vi "EventstringCounter.vi"(3 "error in":errorcluster, 4 "Reset Count":bool, 5 "Increment":bool) -> (0 "error out":errorcluster, 2 "Count":u32)   [LabVIEW 2011]
doc: "Keeps count of anything you want. In this case it is meant to keep track of the number of eventstrings we've sent.\n\nSo you should call this with \"Reset Count\" = TRUE in the initialization code, and then with \"Increment\" = TRUE every time you send an eventstring. Then \"Count\" will return the total number of eventstrings sent.\n\nNo error handling happens; the error in/error out is just to help you sequence your code using dataflow."
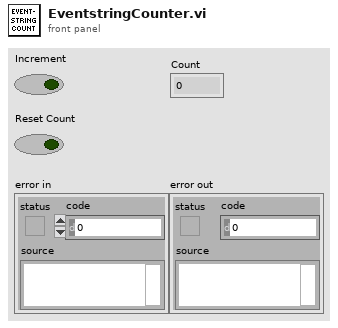
[diagram p1: front panel]
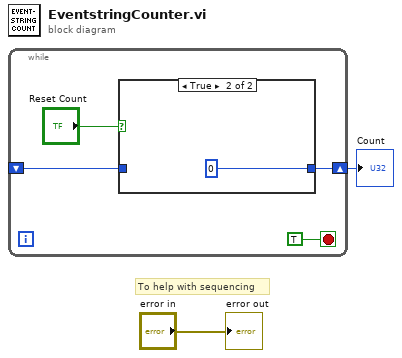
[diagram p0: block diagram]
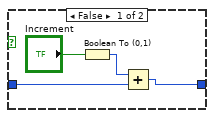
[diagram p2: hidden frame]
diagram:
  # "To help with sequencing"
  n1 = while {
    shift-right: [w4] -> w1
    shift-left: _ -> [w3]
    stop <- TRUE ("stop") stop-if-true
    n2 = case shown="True" "Reset Count" {
      tunnel: [w7 u32 0 ("Count")] -> w4
      tunnel: w3 -> [w8 _]
      frame False {
        n3 = Boolean To (0,1)(Boolean="Increment") -> (0, 1=w9:i16)
        n4 = Add(x=w9, y=w8) -> (x+y=w7:u32)
      }
      frame True {
      }
    }
  }
  "Count" <- w1
  "error out" <- "error in"
